vi "Light On Off.vi"() -> ()   [LabVIEW 2020]
uses:
  5c1df547-9f86-4596-9bc8-9d5d03c6eef4.vi
  Private/Search ID by Name.vi
  Private/Build State URL.vi
  5c1df547-9f86-4596-9bc8-9d5d03c6eef4.vi/f10edee5-3db4-4843-a358-6f175c3e5c4d.vi
  Private/Search ID by Name.vi/3d9aac69-2a40-4ca4-b0c0-ef428fe3223d.vi
  <vilib>/JDP Science/JSONtext/Variant to JSON Text.vi
  <vilib>/httpClient/PUT.vi
  <vilib>/httpClient/PUTBuffer.vi
  LMH-Hue.lvlib
panel:
  in  "Light Name":string="office edison"
  out "error out":errorcluster
  out "Response":string
  in  "Checkbox":bool
  in  "Hostname / IP":string="192.168.1.3"
  in  "Username":string="n2E5i0EwzIpdamkjJWehfzOrC8RPhy6IB12A83ts"
  in  "ID":u8=3
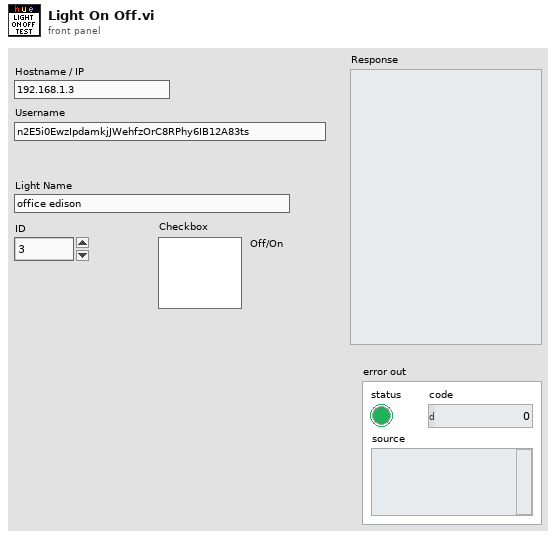
[diagram p1: front panel]
types:
  T1 = typedef "LMH-Hue.lvlib/Hue Ref.ctl" = cluster{"HTTP Session":T2, "Base URL":string, "Map":map{i32, T3}}
  T2 = typedef "LabVIEWHTTPClient.lvlib/ClientHandle.ctl" = refnum<k1>
  T3 = typedef "LMH-Hue.lvlib/Light Data.ctl" = cluster{"Name":string, "On?":bool, "Reachable?":bool, "Color?":bool}
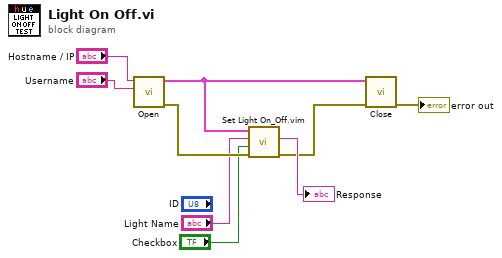
[diagram p0: block diagram]
diagram:
  n1 = call "Open.vi"("Username"="Username", "Hostname / IP"="Hostname / IP") -> ("Error Out"=w8:errorcluster, "Hue Config"=w9:T1)  [unwired: 8 in]
  n2 = call "Set Light On_Off.vim"("error in"=w8, "Light Control"="Checkbox", "ID"="Light Name", "Hue Config"=w9) -> ("error out"=w3:errorcluster, "Response"=→"Response":string)  [unwired: 6 in]
  n3 = call "Close.vi"("Error In"=w3, "Hue Config"=w9) -> ("Error Out"=→"error out":errorcluster)  [unwired: 9 in]
